vi "ACal-Plot Data.vi"(0 "Path":path, 1 "Name":string, 5 "Mag graph":refnum<vi>, 9 "Plot.Line Width":u8=2, 11 "error in (no error)":errorcluster, 12 "Plot max":bool) -> (4 "Path (out)":path, 15 "error out":errorcluster)   [LabVIEW 2020]
doc: "This helper VI loads calibration data from a file, and plots the magnitude and phase on graphs whose references are inputs to the VI. Handles the logic of overplotting data, selecting the colors and linestyles, and inserting the filename into the legend.\n\nKEH 9/10/09"
uses:
  PXI DAQ VIs/DAQ Engine VIs/PXI Globals.vi
  Utility VIs/Math VIs/Linear to dB (scalar).vi
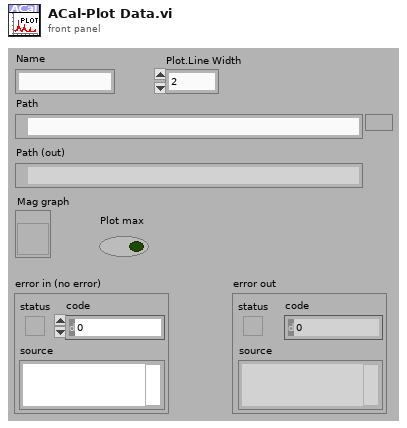
[diagram p1: front panel]
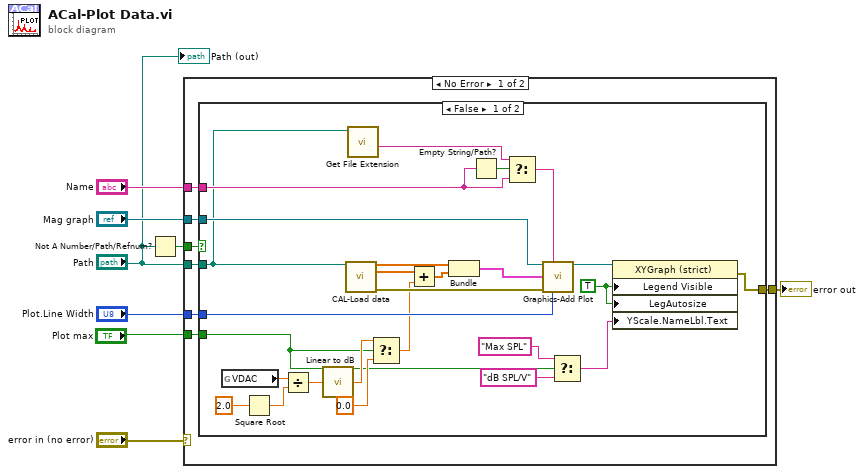
[diagram p0: block diagram]
diagram:
  n1 = Not A Number/Path/Refnum?(number/path/refnum="Path") -> (NaN/Path/Refnum?=w6:bool)
  n2 = case shown="No Error" "error in (no error)" {
    selector: "error in (no error)" -> [_ w42]
    tunnel: "Mag graph" -> [w15 _]
    tunnel: [w10 w42] -> w7
    tunnel: w6 -> [w14 _]
    tunnel: "Path" -> [w13 _]
    tunnel: "Name" -> [w12 _]
    tunnel: "Plot.Line Width" -> [w11 _]
    tunnel: "Plot max" -> [w9 _]
    frame No Error {
      n3 = case shown="False" w14 {
        tunnel: w15 -> [w37 _]
        tunnel: w13 -> [w32 _]
        tunnel: w12 -> [w35 _]
        tunnel: w11 -> [w33 _]
        tunnel: [w29 _] -> w10
        tunnel: w9 -> [w19 _]
        frame False {
          w28 = TRUE ("Legend:Visible")
          n4 = global read "PXI Globals.vi" "VDAC"() -> (w23:dbl)
          n5 = Square Root(x=2.0) -> (sqrt(x)=w24:dbl)
          n6 = Divide(x=w23, y=w24) -> (x/y=w26:dbl)
          n7 = call-poly "Linear to dB.vi"("Linear"=w26) -> ("dB"=w22:dbl)
          n8 = call "CAL-Load data.vi"("user path"=w32) -> ("Frequency (Hz)"=w41:dbl[], "Mag"=w40:dbl[], "error out"=w39:errorcluster)  [unwired: 7 in, 5 out]
          n9 = call <vilib>:"Get File Extension.vi"("file"=w32) -> ("filename without extension"=w31:string)  [unwired: 6 in, 4 out]
          n10 = Select(t=w22, s=w19, f=0.0) -> (s? t:f=w20:dbl)
          n11 = Add(x=w40, y=w20) -> (x+y=w21:dbl[])
          n12 = Bundle("Frequency (Hz)"=w41, w21) -> (w38:cluster{"Frequency (Hz)":dbl[], dbl[]})  [unwired: 1 in]
          n13 = Empty String/Path?(string/path=w35) -> (empty?=w36:bool)
          n14 = Select(t=w31, s=w36, f=w35) -> (s? t:f=w34:string)
          n15 = call "Graphics-Add Plot.vi"("XYGraph in"=w37, "Name"=w34, "XY Data"=w38, "error in (no error)"=w39, "Plot.Line Width"=w33) -> ("XYGraph out"=w30:refnum<vi>)  [unwired: 9 in, 1 out]
          n16 = Select(t="Max SPL", s=w19, f="dB SPL/V") -> (s? t:f=w16:string)
          n17 = property class="XYGraph (strict)"(reference=w30, "Legend Visible"=w28, "LegAutosize"=w28, "YScale.NameLbl.Text"=w16) -> (error out=w29:errorcluster)  [unwired: 1 in, 1 out]
        }
        frame True {
        }
      }
    }
    frame Error {
    }
  }
  "error out" <- w7
  "Path (out)" <- "Path"
